vi "Post-Install Custom Action.vi"(10 "Variant":variant) -> (0 "error out":errorcluster)   [LabVIEW 2015]
uses:
  <vilib>/Palette API/Palette Menu/Public Type Define/Palette type.ctl
  <vilib>/Palette API/Palette Menu/Public Type Define/Item.ctl
  <vilib>/Palette API/Palette Menu/Palette Menu.lvlib
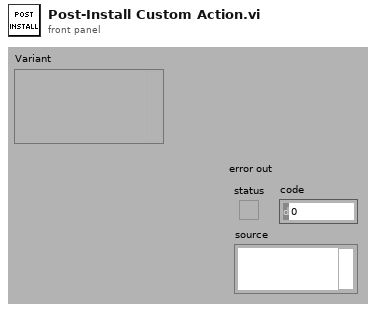
[diagram p1: front panel]
types:
  T1 = typedef "Palette Menu.lvlib/Palette type.ctl" = i32
  T2 = typedef "Palette Menu.lvlib/Palette Data.ctl" = cluster{"display name":string, "view format":T3, "palette width":i16, "items":T4, "256 color icon":picture, "B&W color icon":picture, "help information":T6, "palette description":string, "synchronize information":T7}
  T3 = typedef "Palette Menu.lvlib/View Format.ctl" = u16
  T4 = typedef "Palette Menu.lvlib/Items.ctl" = T5[]
  T5 = typedef "Palette Menu.lvlib/Item.ctl" = cluster{"item path":path, "library path (.lvlib)":path, "use default lvlib palette":bool, "short name":string, "place VI contents":bool, "hide synchronized item":bool, "reserve spot for synch item":bool, "configure when placing VI contents":bool}
  T6 = typedef "Palette Menu.lvlib/Help Info.ctl" = cluster{"help tag":string, "help file path ":path}
  T7 = typedef "Palette Menu.lvlib/Synchronize Info.ctl" = cluster{"synchronize with directory":bool, "synchronize directory path":path}
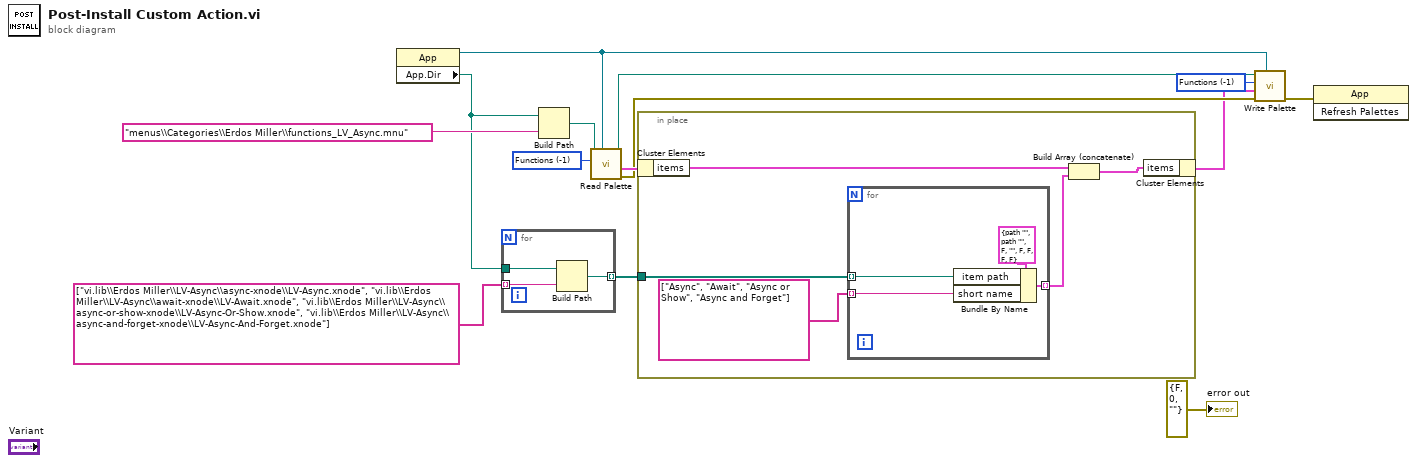
[diagram p0: block diagram]
diagram:
  w6 = T1 -1 items=["Functions"=-1, "Controls"=-2] ("palette type")
  w7 = T1 -1 items=["Functions"=-1, "Controls"=-2] ("palette type")
  n1 = property class="App"() -> (reference out=w8:refnum<vi>, "App.Dir"=w11:path)  [unwired: 2 in, 1 out]
  n2 = for {
    tunnel: string[] ["vi.lib\\Erdos Miller\\LV-Async\\async-xnode\\LV-Async.xnode", "vi.lib\\Erdos Miller\\LV-Async\\await-xnode\\LV-Await.xnode", "vi.lib\\Erdos Miller\\LV-Async\\async-or-show-xnode\\LV-Async-Or-Show.xnode", "vi.lib\\Erdos Miller\\LV-Async\\async-and-forget-xnode\\LV-Async-And-Forget.xnode"] -> [w16] mode=indexing
    tunnel: w11 -> [w17]
    tunnel: [w15] -> w3 mode=indexing
    n3 = Build Path(base path=w17, name or relative path=w16) -> (appended path=w15:path)
  }
  n4 = Build Path(base path=w11, name or relative path="menus\\Categories\\Erdos Miller\\functions_LV_Async.mnu") -> (appended path=w2:path)
  n5 = call <vilib>:"Read Palette.vi"("application reference"=w8, "palette type"=w6, "palette path"=w2) -> ("error out"=w9:errorcluster, "palette data"=w12:T2, "duplicate palette path"=w10:path)  [unwired: 6 in]
  n6 = in-place {
    in-place-border: w3 -> [w22]
    n7 = in-place-cluster #1(w12) -> ("items"=w21:T4)
    n8 = for {
      tunnel: w22 -> [w25] mode=indexing
      tunnel: [w24] -> w20 mode=indexing
      tunnel: string[] ["Async", "Await", "Async or Show", "Async and Forget"] -> [w23] mode=indexing
      n9 = Bundle By Name(cluster=T5 {"item path"=path "", "library path (.lvlib)"=path "", "use default lvlib palette"=FALSE, "short name"="", "place VI contents"=FALSE, "hide synchronized item"=FALSE, "reserve spot for synch item"=FALSE, "configure when placing VI contents"=FALSE} ("Items"), "item path"=w25, "short name"=w23) -> (w24:T5)
    }
    n10 = Build Array (concatenate)(w21, w20) -> (w19:T4)
    n11 = in-place-cluster #1("items"=w19) -> (w4:T2)
  }
  n12 = call <vilib>:"Write Palette.vi"("application reference"=w8, "error in (no error)"=w9, "palette data"=w4, "palette type"=w7, "palette path"=w10) -> ("error out"=w5:errorcluster)  [unwired: 6 in]
  n13 = invoke class="App" method="Refresh Palettes"(error in=w5) -> ()  [unwired: 2 in, 3 out]
  "error out" <- errorcluster {"status"=FALSE, "code"=0, "source"=""} ("error out")
